vi "Double_word_to_real_float.vi"(9 "Seconda WORD":u16, 11 "Prima WORD":u16) -> (3 "Real float":dbl format="%#.6f")   [LabVIEW 2022 SP3]
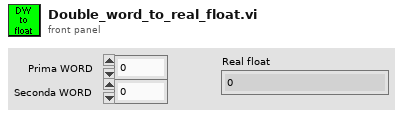
[diagram p1: front panel]
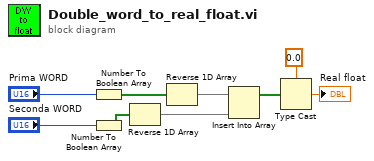
[diagram p0: block diagram]
diagram:
  n1 = Number To Boolean Array(number="Prima WORD") -> (Boolean array=w6:bool[])
  n2 = Number To Boolean Array(number="Seconda WORD") -> (Boolean array=w5:bool[])
  n3 = Reverse 1D Array(array=w5) -> (reversed array=w3:bool[])
  n4 = Reverse 1D Array(array=w6) -> (reversed array=w4:bool[])
  n5 = Insert Into Array(array=w4, new element=w3) -> (w2:bool[])  [unwired: 1 in]
  n6 = Type Cast(type=sgl 0.0 ("V_TEMP_AMBIENTE 3"), x=w2) -> (*(type *) &x=→"Real float":sgl)
